vi "GetBoolean.vi"(6 "false string (0)":string="0", 7 "key description":string, 8 "sections":string[](array[string]), 9 "boolean":bool, 11 "info data":string) -> (0 "sections out":string[](array[string]), 1 "key found?":bool, 2 "value":bool, 3 "info data out":string)   [LabVIEW 2013, in "infolib.lvlib"]
doc: "Add a new numeric key to Info Data string. If section exists in Info Data string, inserts key into this section."
uses:
  infolib.lvlib
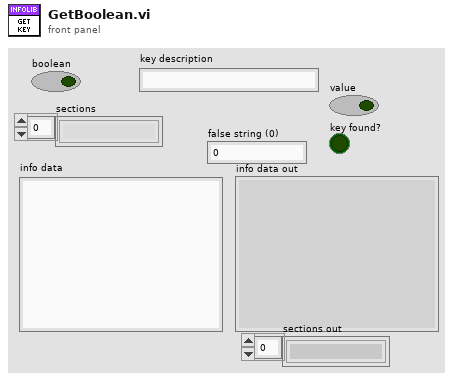
[diagram p1: front panel]
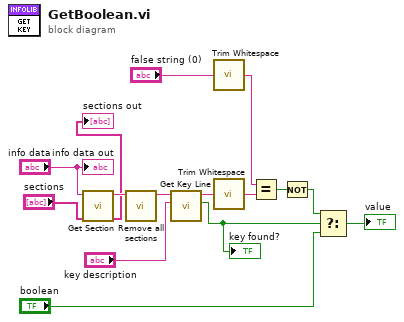
[diagram p0: block diagram]
diagram:
  n1 = call "Get Section.vi"("sections"="sections", "info data"="info data") -> ("sections out"=→"sections out":string[], "section part"=w15:string)  [unwired: 7 in, 1 out]
  n2 = call "Remove all sections.vi"("info data"=w15) -> ("info data out"=w14:string)  [unwired: 10 in]
  n3 = call "Get Key Line.vi"("key description"="key description", "info data"=w14) -> ("key found?"=w1:bool, "key value"=w8:string)  [unwired: 8 in]
  "key found?" <- w1
  n4 = call <vilib>:"Trim Whitespace.vi"("string"="false string (0)") -> ("trimmed string"=w10:string)  [unwired: 1 in]
  n5 = call <vilib>:"Trim Whitespace.vi"("string"=w8) -> ("trimmed string"=w9:string)  [unwired: 1 in]
  n6 = Equal?(x=w10, y=w9) -> (x = y?=w7:bool)
  n7 = Not(x=w7) -> (.not. x?=w4:bool)
  n8 = Select(t=w4, s=w1, f="boolean") -> (s? t:f=→"value":bool)
  "info data out" <- "info data"
